vi "p1.vi"() -> ()   [LabVIEW 2023, in "d14.lvlib"]
uses:
  d14.lvlib
  AOC/AOC.lvlib
panel:
  out "Answer":i32
  in  "Example":string
  in  "Example":bool
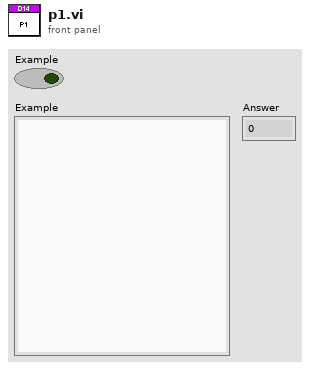
[diagram p1: front panel]
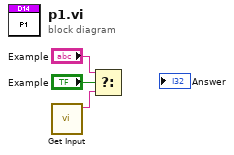
[diagram p0: block diagram]
diagram:
  n1 = call "Get Input.vi"() -> ("Input"=w3:string)  [unwired: 11 in]
  n2 = Select(t="Example", s="Example", f=w3) -> ()  [unwired: 1 out]
